vi "Read Channel Info.vi"(8 "error in (no error)":errorcluster, 11 "Readable.lvclass in":refnum<class "Readable.lvclass">) -> (0 "error out":errorcluster, 1 "Channel Units":T1, 2 "Channel Names":T2, 3 "Readable.lvclass out":refnum<class "Readable.lvclass">, 5 "#Channels":i32)   [LabVIEW 2015, in "Readable.lvclass"]
doc: "(Dynamic) Return information about the readable data channels this object provides, e.g., the name of each data source and its unit."
uses:
  Readable.lvclass
  Channel Names.ctl
  Channel Units.ctl
  Readable.lvclass/Readable.ctl
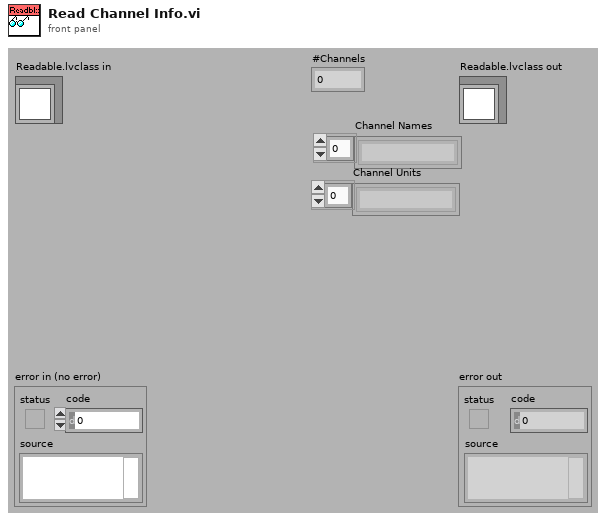
[diagram p1: front panel]
types:
  T1 = typedef "Readable.lvclass/Channel Units.ctl" = string[]
  T2 = typedef "Readable.lvclass/Channel Names.ctl" = string[]
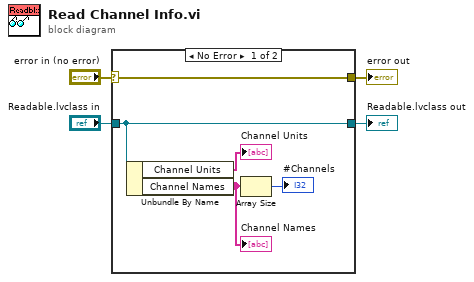
[diagram p0: block diagram]
diagram:
  n1 = case shown="No Error" "error in (no error)" {
    selector: "error in (no error)" -> [w8 w10]
    tunnel: [w8 w10] -> w3
    tunnel: [w6 w11] -> w1
    tunnel: "Readable.lvclass in" -> [w6 w11]
    frame No Error {
      n2 = Unbundle By Name(w6) -> ("Channel Units"=→"Channel Units":T1, "Channel Names"=w5:T2)
      "Channel Names" <- w5
      n3 = Array Size(array=w5) -> (size(s)=→"#Channels":i32)
    }
    frame Error {
    }
  }
  "error out" <- w3
  "Readable.lvclass out" <- w1
